vi "SetExternalInterfaces.vi"(8 "ErrorIn":errorcluster, 10 "ExternalInterfaces":T1[](array[typedef]), 11 "ReferenceIn":refnum<class "DemoApplication.lvclass">) -> (0 "ErrorOut":errorcluster, 3 "ReferenceOut":refnum<class "DemoApplication.lvclass">)   [LabVIEW 2021, in "DemoApplication.lvclass"]
uses:
  DemoApplication.lvclass
  .Externals/Library_TAF_Support/ClusterArrayConversion/BundledArray.ctl
  23b01655-c9ef-4a3c-a018-7f9b77e1bca9.vi
  0a6ec689-4898-488c-8e07-ed5616c8d135.vi
  0a6ec689-4898-488c-8e07-ed5616c8d135.vi/e733eca7-9823-4359-8665-3b184f9a7377.vi
  0a6ec689-4898-488c-8e07-ed5616c8d135.vi/185eb5ab-e8f7-4395-854b-f566a9b9020c.vi
  <vilib>/Utility/Data Type/Get Cluster Information.vi
  <vilib>/Utility/Data Type/Get Type Information.vi
  <userlib>/_OpenG.lib/lvdata/lvdata.llb/Array of VData to VCluster__ogtk.vi
  <vilib>/Utility/LVClass/Get LV Class Name.vi
  .Externals/Library_TAF_ApplicationFramework/MasterGUI/MasterGUI.lvclass
  .Externals/Library_TAF_Support/ClusterArrayConversion/ClusterArrayConversion.lvlib
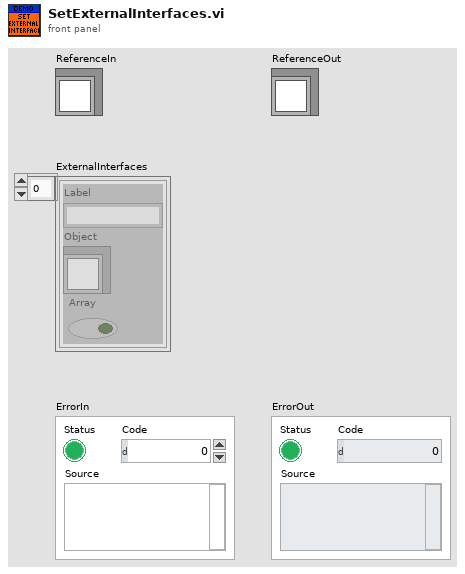
[diagram p1: front panel]
types:
  T1 = typedef "ClusterArrayConversion.lvlib/BundledArray.ctl" = cluster{"Label":string, "Object":refnum<class>, "Array":bool}
  T2 = typedef "DemoApplication.lvclass/ObjectAttributes.ctl" = cluster{"Interfaces":cluster{"Authorizer":refnum<class "IAuthorization.lvclass">, "TextViewer":refnum<class "ITAFTextViewer.lvclass">, "ApplicationConfiguration":refnum<class "IApplicationConfiguration.lvclass">, "Tracer":refnum<class "IFrontPanel.lvclass">}, "Persistent":cluster{"MenuEnables":cluster{"MenuTag":string, "MenuExpression":string}[], "TextDockSubPanelName":string}}
  T3 = cluster{"Authorizer":refnum<class "IAuthorization.lvclass">, "TextViewer":refnum<class "ITAFTextViewer.lvclass">, "ApplicationConfiguration":refnum<class "IApplicationConfiguration.lvclass">, "Tracer":refnum<class "IFrontPanel.lvclass">}
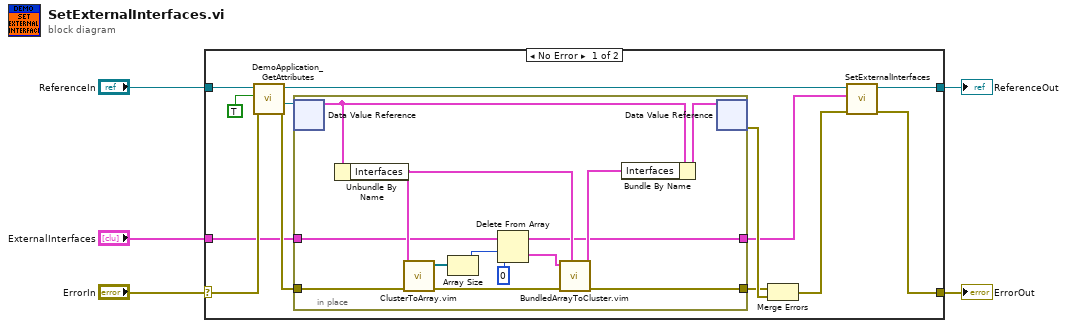
[diagram p0: block diagram]
diagram:
  n1 = case shown="No Error" "ErrorIn" {
    selector: "ErrorIn" -> [w18 w33]
    tunnel: [w13 w33] -> w4
    tunnel: [w7 w32] -> w2
    tunnel: "ReferenceIn" -> [w12 w32]
    tunnel: "ExternalInterfaces" -> [w9 _]
    frame No Error {
      n2 = call "DemoApplication_GetAttributes.vi"("ErrorIn"=w18, "OnlyGetDvrReference(False)"=TRUE, "ReferenceIn"=w12) -> ("ErrorOut"=w15:errorcluster, "DataRef"=w10:refnum<data-value>, "ReferenceOut"=w8:refnum<class "DemoApplication.lvclass">)  [unwired: 5 in, 1 out]
      n3 = in-place {
        in-place-border: [w31] -> w16
        in-place-border: w15 -> [w30]
        in-place-border: w9 -> [w24]
        in-place-border: [w19] -> w6
        n4 = in-place-dvr #1(w10) -> (w27:T2)  [unwired: 1 out]
        n5 = Unbundle By Name(w27) -> ("Interfaces"=w25:T3)
        n6 = call "ClusterToArray.vim"("ErrorIn"=w30, "Cluster"=w25) -> ("ErrorOut"=w29:errorcluster, "ArrayOfElements"=w22:refnum<class "IInterface.lvclass">[])  [unwired: 7 in, 1 out]
        n7 = Array Size(array=w22) -> (size(s)=w21:i32)
        n8 = Delete From Array(array=w24, length=w21, index=0) -> (deleted portion=w23:T1[], array with subset deleted=w19:T1[])
        n9 = call "BundledArrayToCluster.vim"("Type"=w25, "ErrorIn"=w29, "BundeledLabels"=w23) -> ("ErrorOut"=w31:errorcluster, "DataOut"=w26:T3)  [unwired: 7 in]
        n10 = Bundle By Name(cluster=w27, "Interfaces"=w26) -> (w28:T2)
        n11 = in-place-dvr #1(w28) -> (w17:errorcluster)  [unwired: 1 out]
      }
      n12 = Merge Errors(w16, w17) -> (w14:errorcluster)
      n13 = call-parent "SetExternalInterfaces.vi"("ErrorIn"=w14, "ExternalInterfaces"=w6, "ReferenceIn"=w8) -> ("ErrorOut"=w13:errorcluster, "ReferenceOut"=w7:refnum<class "DemoApplication.lvclass">)  [unwired: 7 in]
    }
    frame Error {
    }
  }
  "ErrorOut" <- w4
  "ReferenceOut" <- w2
